vi "GlobalTempHum.vi"() -> ()   [LabVIEW 2024]
panel:
  out "Temp/Hum":string
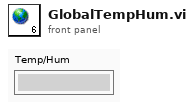
[diagram p1: front panel]
diagram:
